vi "Main2.vi"() -> ()   [LabVIEW 2013]
uses:
  controls/Microprobe Vars.ctl
  <userlib>/SweepParameters.ctl
  controls/State.ctl
  controls/ProgramState.ctl
  <instrlib>/Watlow EZ-ZONE/Public/Watlow_Set_Parameter.ctl
  <instrlib>/IMS stepper motors/Address.ctl
  <instrlib>/IMS stepper motors/Set Parameter.ctl
  controls/ProgramColumn.ctl
panel:
  in  "Probe Target State":T1 {"Tset" format="%.1f"; "Telem" format="%.1f"; "GasC" format="%.1f"; "GasB" format="%.1f"; "GasA" format="%.1f"; "Z" format="%.3g"; "Y" format="%.3g"; "X" format="%.3g"; "RampRate" format="%.1f"}
  out "Probe Current State":T1 {"Tset" format="%.1f"; "Telem" format="%.1f"; "GasC" format="%.1f"; "GasB" format="%.1f"; "GasA" format="%.1f"; "Z" format="%.3g"; "Y" format="%.3g"; "X" format="%.3g"; "RampRate" format="%.1f"}
  in  "Exit":bool
  in  "Tab Control":T2(tab)
  in  "Gas B pO2":dbl=0.001
  in  "Gas A pO2":dbl=0.2
  in  "Sample name":string="ZDC30TG3"
  in  "Impedance analyzer":refnum<visa-resource-name>="GPIB0::17::INSTR"
  out "Test sequence path":path
  out "Log file path":path
  out "Sample directory":path
  in  "Motor":refnum<visa-resource-name>="COM9"
  in  "Temp controller":refnum<visa-resource-name>="COM3"
  in  "MFCs":refnum<visa-resource-name>="COM5"
  in  "Inert MFC address":i32=8
  in  "Active MFC address":i32=7
  in  "Instrument type":T3(ring)=enum."BioLogic SP-300"
  out "Estimated pO2":dbl
  in  "Set current as origin":bool
  out "Temperature vs time":dbl(graph)
  in  "Jog to Y":dbl format="%.3g"
  in  "Jog to X":dbl format="%.3g"
  in  "Jog":bool
  out "Chiller flow?":bool
  out "Gases vs time":cluster{"GasA":dbl, "GasB":dbl, "GasC":dbl}(graph)
  out "State":T4
  in  "Run program":bool
  in  "Program":string[][](table)
  in  "Read program":bool
  out "Program data":dbl[][](array[numeric])
  out "Cur step":i32
  in  "Start step":i32=1
  out "Number of steps":i32
  out "Est. time":dbl
  out "Program state":T5
  out "Waiting":dbl
  in  "Take single AC Scan":bool
  in  "Sweep Parameters":T6={"Frequency steps"=41, "Sweep Direction"=enum."Down", "Max frequency (Hz)"=1000000.0, "Min frequency (Hz)"=100.0, "Voltage Level (V)"=0.03, "bias(V)"=0.0} {"Voltage Level (V)" min=0.005 max=20.0 step=0.001 format="%.4f"; "Min frequency (Hz)" format="%#_6e"; "Max frequency (Hz)" format="%#_6e"}
  out "Impedance plot":cluster{dbl[], dbl[]}(graph)
  in  "check if\ntouching\nparams":T6={"Frequency steps"=6, "Sweep Direction"=enum."Down", "Max frequency (Hz)"=1000.0, "Min frequency (Hz)"=100.0, "Voltage Level (V)"=0.03, "bias(V)"=0.0} {"Voltage Level (V)" min=0.005 max=20.0 step=0.001 format="%.4f"; "Min frequency (Hz)" format="%#_6e"; "Max frequency (Hz)" format="%#_6e"}
  out "error out":errorcluster
  out "Monitoring error":errorcluster
  out "State machine error":errorcluster
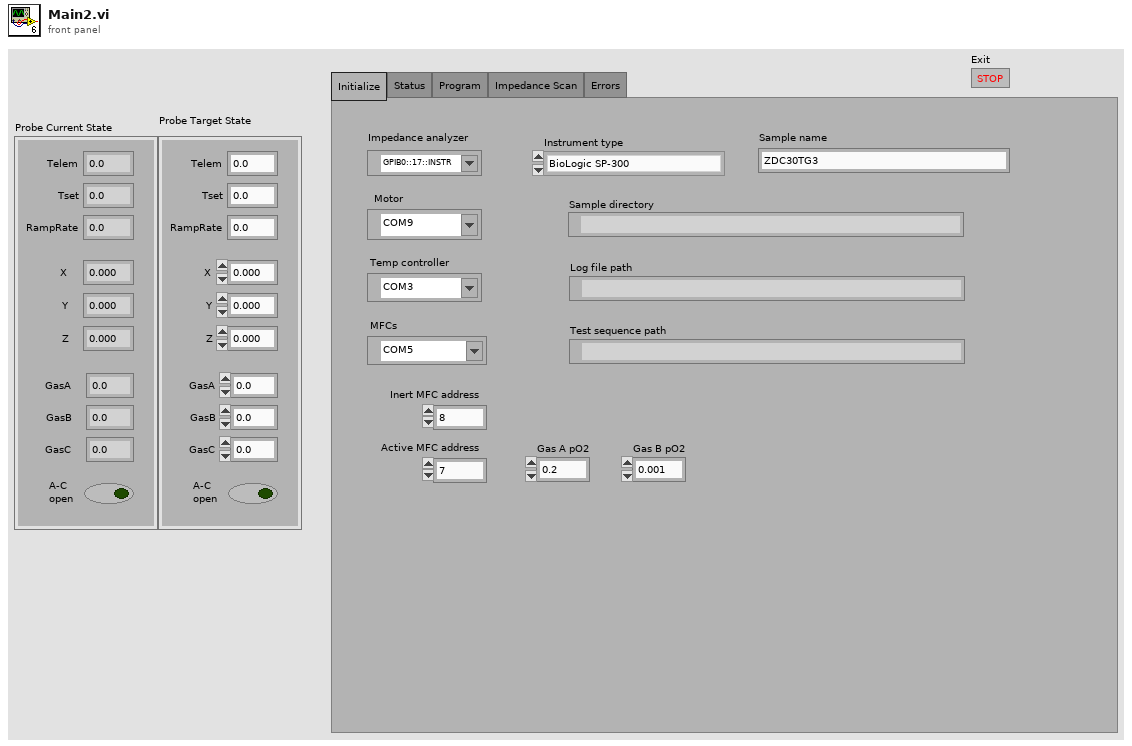
[diagram p1: front panel]
types:
  T1 = typedef "Microprobe Vars.ctl" = cluster{"Telem":dbl, "Tset":dbl, "RampRate":dbl, "X":dbl, "Y":dbl, "Z":dbl, "GasA":dbl, "GasB":dbl, "GasC":dbl, "A-C\nopen":bool}
  T2 = enum32{"Initialize", "Status", "Program", "Impedance Scan", "Errors"}
  T3 = enum16{"Agilent 4285A", "Solartron 1260", "BioLogic SP-300"}
  T4 = typedef "State.ctl" = enum16{"Idle", "Jog", "Run AC Scan", "Run Program", "Exit"}
  T5 = typedef "ProgramState.ctl" = enum16{"Lift Z", "Read program", "Set gas", "Set temperature", "Wait for temperature", "Delay", "Check if running", "Move to position", "Check if touching", "Wait for measurement", "Take measurement", "Move away", "Move to next step?"}
  T6 = typedef "SweepParameters.ctl" = cluster{"Frequency steps":i32, "Sweep Direction":enum16{"Down", "Up"}, "Max frequency (Hz)":dbl, "Min frequency (Hz)":dbl, "Voltage Level (V)":dbl, "bias(V)":dbl}
  T7 = typedef "Watlow_Set_Parameter.ctl" = enum16{"Setpoint", "Ramp Rate", "Setpoint Min", "Setpoint Max"}
  T8 = typedef "Address.ctl" = enum16{"X", "Y", "Z"}
  T9 = typedef "Set Parameter.ctl" = enum16{"Acceleration (A)", "Baud Rate (BD)", "Counter 1 (C1)", "Counter 2 (C2)", "Control C Software Reset (CE)", "Check Sum Enable (CK)", "Clock Mode (CM)", "Clock Mode Ratio (CR)", "Clock Mode Out Step Width (CW)", "Deceleration (D)", "Digital Filtering, Input 1 (D1)", "Digital Filtering, Input 2 (D2)", "Digital Filtering, Input 3 (D3)", "Digital Filtering, Input 4 (D4)", "Digital Filtering, Input 5 (D5)", "Digital Filtering, Input 9 (D9)", "Digital Filtering, Input 10 (D10)", "Digital Filtering, Input 11 (D11)", "Digital Filtering, Input 12 (D12)", "Deadband (DB)", "Decrement Variable (DC)", "Enable/Disable Drive (DE)", "Device Name (DN)", "End Program Execution (E)", "Encoder Function Enable (EE)", "Encoder Lines (EL)", "Echo Mode (EM)", "Escape (ES)", "Execute Program at Address (EX)", "Hold (H)", "Hold Current (HC)", "Hold Current Delay Time (HI)", "Home to Encoder Index (HM)", "Home to Home Switch (HT)", "Increment Variable (IC)", "Initialize Parameters to NVM (IP)", "Input into Variable (IV)", "Jog Enable (JE)", "Limit Stop Mode (LM)", "Move Absolute (MA)", "Move Relative (MR)", "MicroStepping Select (MS)", "Motor Settling Delay Time (MT)", "Output 1 (O1)", "Output 2 (O2)", "Output 3 (O3)", "Output 4 (O4)", "Output 9 (O9)", "Output 10 (O10)", "Output 11 (O11)", "Output 12 (O12)", "Output High Byte (9-12) (OH)", "Output Low Byte (1-4) (OL)", "Output Total (1-4 and 9-12) (OT)", "Position Maintenance (PM)", "Party Mode (PY)", "Register 1 (R1)", "Register 2 (R2)", "Register 3 (R3)", "Register 4 (R4)", "Run Current (RC)", "SetupLimits (S1,S2)", "Stall Factor (SF)", "Slew (SL)", "Stall Mode Set (SM)", "Upgrade Firmware (UG)", "Velocity Initial (VI)", "Velocity Maximum (VM)"}
  T10 = typedef "ProgramColumn.ctl" = enum16{"Run Number", "Stage Temperature", "Ramp Rate", "Wait", "Gas A", "Gas B", "Gas C", "Row index I", "Column index J", "X position", "Y position", "Z position", "Voltage", "Highest frequency", "Lowest frequency", "Number of freq pts", "Delay", "Move this step?", "bias(V)"}
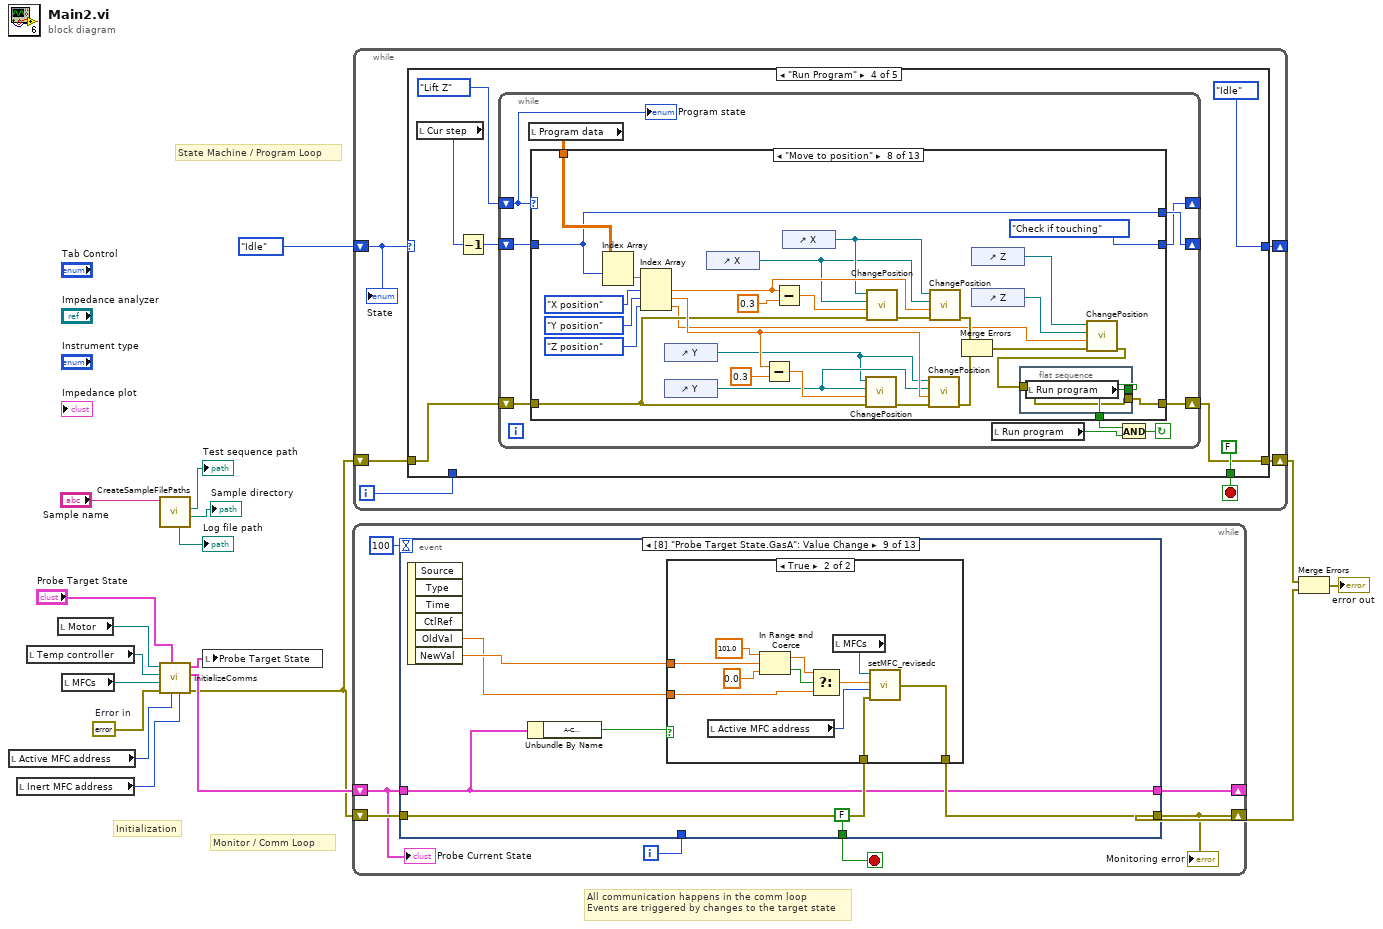
[diagram p0: block diagram]
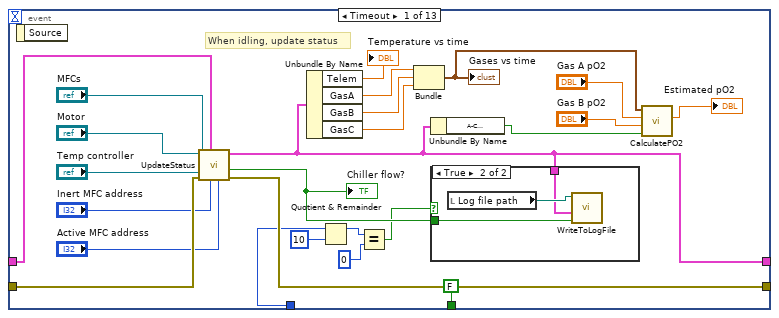
[diagram p2: hidden frame]
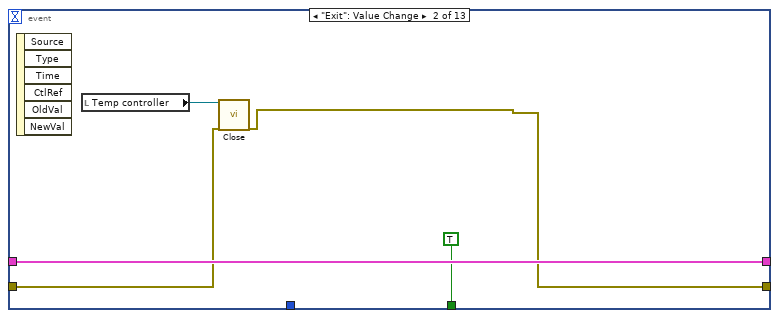
[diagram p4: hidden frame]
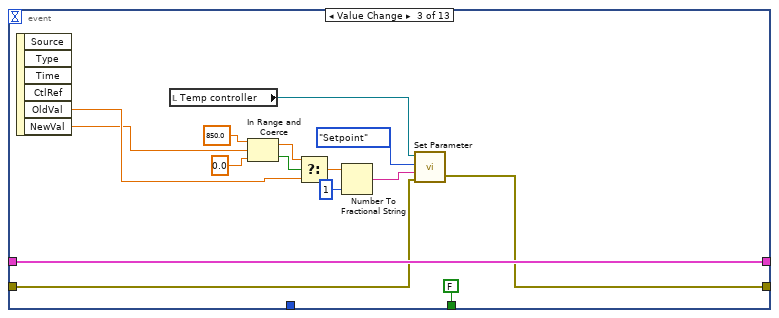
[diagram p5: hidden frame]
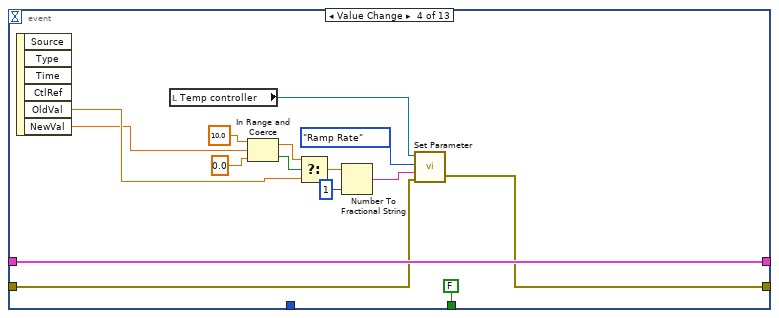
[diagram p6: hidden frame]
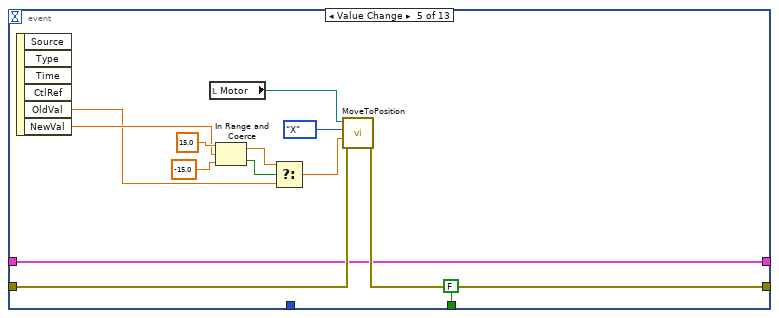
[diagram p7: hidden frame]
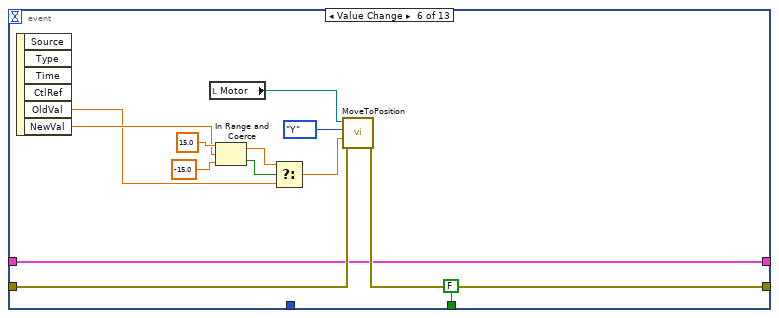
[diagram p8: hidden frame]
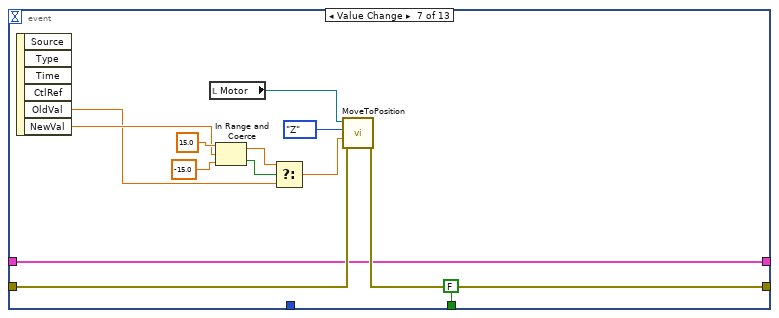
[diagram p9: hidden frame]
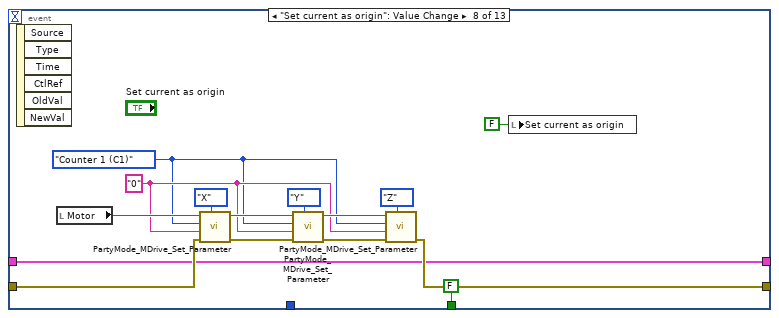
[diagram p10: hidden frame]
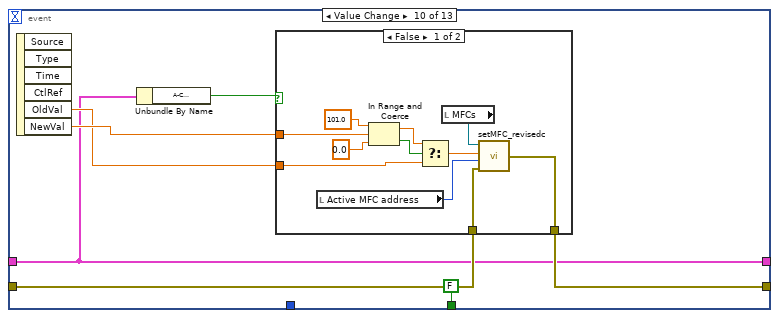
[diagram p12: hidden frame]
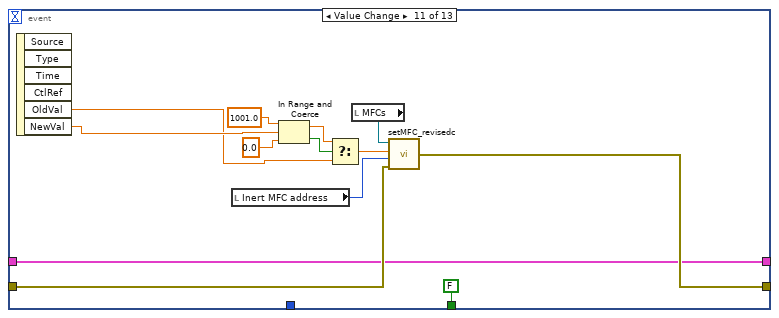
[diagram p14: hidden frame]
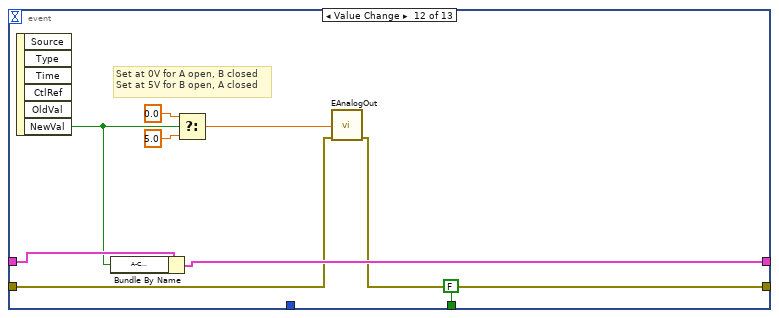
[diagram p15: hidden frame]
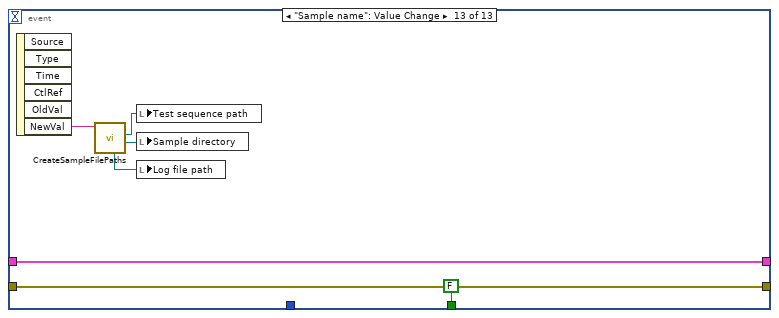
[diagram p16: hidden frame]
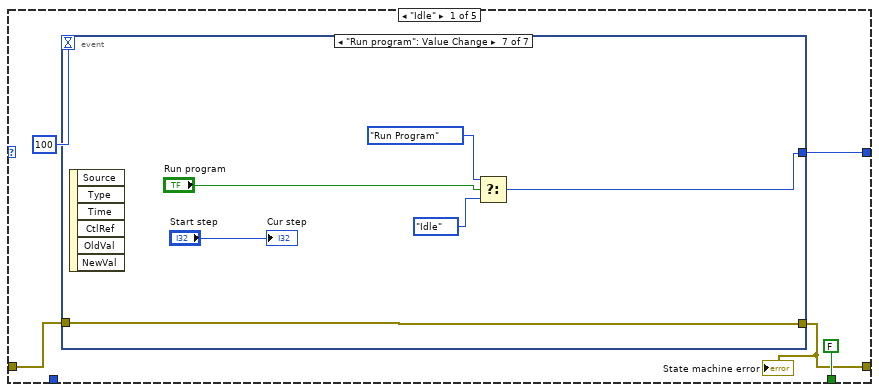
[diagram p17: hidden frame]
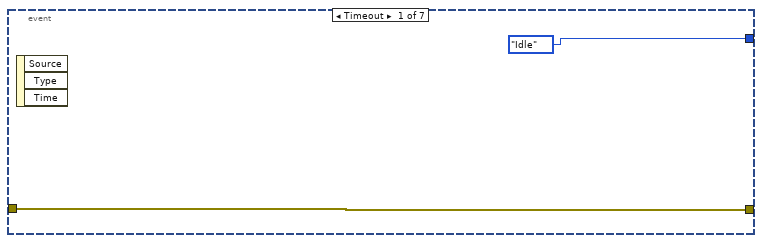
[diagram p18: hidden frame]
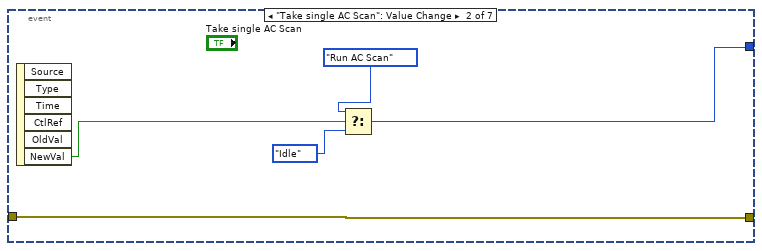
[diagram p19: hidden frame]
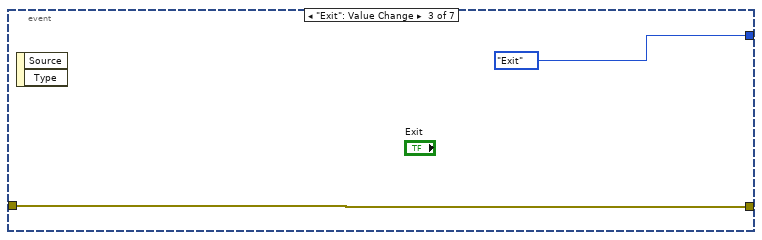
[diagram p20: hidden frame]
diagram:
  w3 = errorcluster {"status"=FALSE, "code"=0, "source"=""}  # Error in
  # "All communication happens in the comm loop\nEvents are triggered by changes to the target state"
  # "Initialization"
  # "State Machine / Program Loop"
  # "Monitor / Comm Loop"
  n1 = local read "Active MFC address"() -> (w8:i32)
  n2 = local read "Inert MFC address"() -> (w7:i32)
  n3 = local read "Temp controller"() -> (w10:refnum<visa-resource-name>)
  n4 = local read "Motor"() -> (w11:refnum<visa-resource-name>)
  n5 = local read "MFCs"() -> (w9:refnum<visa-resource-name>)
  n6 = call "CreateSampleFilePaths.vi"("Sample name"="Sample name") -> ("Sample directory path"=→"Sample directory":path, "Test sequence path"=→"Test sequence path":path, "Log file path"=→"Log file path":path)  [unwired: 8 in]
  n7 = call "InitializeComms.vi"("Inert MFC Channel"=w7, "Active MFC Channel"=w8, "Probe Target State"="Probe Target State", "error in"=w3, "MFC channel"=w9, "Watlow channel"=w10, "Motor channel"=w11) -> ("error out"=w1:errorcluster, "Current probe state"=w6:T1, "Probe Target State out"=w4:T1)  [unwired: 2 in]
  n8 = local write "Probe Target State"(w4) -> ()
  n9 = while {
    shift-right: [w22] -> _
    shift-left: w6 -> [w23]
    shift-right: [w24] -> w16
    shift-left: w1 -> [w25]
    i -> [w19]
    stop <- w20 stop-if-true
    n10 = event shown="[8] \"Probe Target State.GasA\": Value Change" {
      selector: _ -> [_ _ _ _ _ _ _ _ _ _ _ _ _]
      dyn-events: _ -> [_ _ _ _ _ _ _ _ _ _ _ _ _]
      timeout: 100 -> [_ _ _ _ _ _ _ _ _ _ _ _ _]
      tunnel: w25 -> [w46 w56 w61 w76 w100 w113 w126 w141 w147 w166 w185 w195 w205]
      tunnel: [w43 w54 w60 w75 w99 w112 w125 w135 w146 w165 w184 w194 w205] -> w24
      tunnel: w23 -> [w45 w58 w72 w87 w98 w111 w124 w134 w145 w164 w183 w200 w209]
      tunnel: [w32 w58 w72 w87 w98 w111 w124 w134 w145 w164 w183 w199 w209] -> w22
      tunnel: [FALSE TRUE FALSE FALSE FALSE FALSE FALSE FALSE FALSE FALSE FALSE FALSE FALSE] -> w20
      tunnel: w19 -> [w36 _ _ _ _ _ _ _ _ _ _ _ _]
      event Timeout {
        # "When idling, update status"
        n11 = event-data() -> ()  [unwired: 1 in, 1 out]
        n12 = call "UpdateStatus.vi"("Active MFC address"="Active MFC address", "Inert MFC address"="Inert MFC address", "Probe Current State"=w45, "error in"=w46, "MFC Channel"="MFCs", "Watlow channel"="Temp controller", "Motor channel"="Motor") -> ("error out"=w43:errorcluster, "Chiller flow?"=w38:bool, "Updated probe state"=w32:T1)  [unwired: 2 in]
        "Chiller flow?" <- w38
        n13 = Unbundle By Name(w32) -> ("Telem"=→"Temperature vs time":dbl, "GasA"=w40:dbl, "GasB"=w31:dbl, "GasC"=w39:dbl)
        n14 = Quotient & Remainder(x=w36, y=10) -> (x-y*floor(x/y)=w33:i32)  [unwired: 1 out]
        n15 = Equal?(x=w33, y=0) -> (x = y?=w37:bool)
        n16 = Bundle("GasA"=w40, "GasB"=w31, "GasC"=w39) -> (w26:cluster{"GasA":dbl, "GasB":dbl, "GasC":dbl})  [unwired: 1 in]
        "Gases vs time" <- w26
        n17 = Unbundle By Name(w32) -> ("A-C\nopen"=w30:bool)
        n18 = case shown="True" w37 {
          tunnel: w32 -> [_ w52]
          tunnel: w38 -> [_ w51]
          frame False {
          }
          frame True {
            n19 = local read "Log file path"() -> (w53:path)
            n20 = call <instrlib>:"WriteToLogFile.vi"("Chiller flow?"=w51, "Probe Current State"=w52, "file path (dialog if empty)"=w53) -> ()  [unwired: 9 in]
          }
        }
        n21 = call "CalculatePO2.vi"("A-C open"=w30, "Gas B pO2"="Gas B pO2", "Gas A pO2"="Gas A pO2", "Gases vs time"=w26) -> ("Estimated pO2"=→"Estimated pO2":dbl)  [unwired: 7 in]
      }
      event "Exit": Value Change {
        n22 = event-data() -> ()  [unwired: 1 in, 6 out]
        n23 = local read "Temp controller"() -> (w55:refnum<visa-resource-name>)
        n24 = call <instrlib>:"Close.vi"("PC Comms Port"=w55, "Error In"=w56) -> ("Error Out"=w54:errorcluster)  [unwired: 16 in, 1 out]
      }
      event Value Change {
        n25 = event-data() -> ("OldVal"=w63:dbl, "NewVal"=w62:dbl)  [unwired: 1 in, 4 out]
        n26 = local read "Temp controller"() -> (w59:refnum<visa-resource-name>)
        n27 = In Range and Coerce(upper limit=850.0, x=w62, lower limit=0.0) -> (coerced(x)=w71:dbl, In Range?=w66:bool)
        n28 = Select(t=w71, s=w66, f=w63) -> (s? t:f=w70:dbl)
        n29 = Number To Fractional String(number=w70, precision (6)=i16 1) -> (F-format string=w69:string)  [unwired: 2 in]
        n30 = call <instrlib>:"Set Parameter.vi"("Error In"=w61, "Set Parameter"=Watlow_Set_Parameter."Setpoint", "Write Value"=w69, "PC Comms Port"=w59) -> ("Error Out"=w60:errorcluster)  [unwired: 1 out]
      }
      event Value Change {
        n31 = event-data() -> ("OldVal"=w78:dbl, "NewVal"=w77:dbl)  [unwired: 1 in, 4 out]
        n32 = local read "Temp controller"() -> (w74:refnum<visa-resource-name>)
        n33 = In Range and Coerce(upper limit=10.0, x=w77, lower limit=0.0) -> (coerced(x)=w86:dbl, In Range?=w81:bool)
        n34 = Select(t=w86, s=w81, f=w78) -> (s? t:f=w85:dbl)
        n35 = Number To Fractional String(number=w85, precision (6)=i16 1) -> (F-format string=w84:string)  [unwired: 2 in]
        n36 = call <instrlib>:"Set Parameter.vi"("Error In"=w76, "Set Parameter"=Watlow_Set_Parameter."Ramp Rate", "Write Value"=w84, "PC Comms Port"=w74) -> ("Error Out"=w75:errorcluster)  [unwired: 1 out]
      }
      event Value Change {
        n37 = event-data() -> ("OldVal"=w91:dbl, "NewVal"=w94:dbl)  [unwired: 1 in, 4 out]
        n38 = local read "Motor"() -> (w89:refnum<visa-resource-name>)
        n39 = In Range and Coerce(upper limit=15.0, x=w94, lower limit=-15.0) -> (coerced(x)=w92:dbl, In Range?=w93:bool)
        n40 = Select(t=w92, s=w93, f=w91) -> (s? t:f=w90:dbl)
        n41 = call <instrlib>:"MoveToPosition.vi"("error out 2"=w100, "Position"=w90, "Address"=Address."X", "Motor channel"=w89) -> ("error out"=w99:errorcluster)  [unwired: 5 in, 2 out]
      }
      event Value Change {
        n42 = event-data() -> ("OldVal"=w104:dbl, "NewVal"=w107:dbl)  [unwired: 1 in, 4 out]
        n43 = local read "Motor"() -> (w102:refnum<visa-resource-name>)
        n44 = In Range and Coerce(upper limit=15.0, x=w107, lower limit=-15.0) -> (coerced(x)=w105:dbl, In Range?=w106:bool)
        n45 = Select(t=w105, s=w106, f=w104) -> (s? t:f=w103:dbl)
        n46 = call <instrlib>:"MoveToPosition.vi"("error out 2"=w113, "Position"=w103, "Address"=Address."Y", "Motor channel"=w102) -> ("error out"=w112:errorcluster)  [unwired: 5 in, 2 out]
      }
      event Value Change {
        n47 = event-data() -> ("OldVal"=w117:dbl, "NewVal"=w120:dbl)  [unwired: 1 in, 4 out]
        n48 = local read "Motor"() -> (w115:refnum<visa-resource-name>)
        n49 = In Range and Coerce(upper limit=15.0, x=w120, lower limit=-15.0) -> (coerced(x)=w118:dbl, In Range?=w119:bool)
        n50 = Select(t=w118, s=w119, f=w117) -> (s? t:f=w116:dbl)
        n51 = call <instrlib>:"MoveToPosition.vi"("error out 2"=w126, "Position"=w116, "Address"=Address."Z", "Motor channel"=w115) -> ("error out"=w125:errorcluster)  [unwired: 5 in, 2 out]
      }
      event "Set current as origin": Value Change {
        w132 = Set_Parameter."Counter 1 (C1)" ("Set Parameter")
        w133 = "0" ("Parameter Setpoint")
        n52 = event-data() -> ()  [unwired: 1 in, 6 out]
        n53 = local read "Motor"() -> (w138:refnum<visa-resource-name>)
        n54 = call <instrlib>:"PartyMode_MDrive_Set_Parameter.vi"("Address"=Address."X", "error out 2"=w141, "Parameter Setpoint"=w133, "Set Parameter"=w132, "VISA resource name out 2"=w138) -> ("error out"=w140:errorcluster, "VISA resource name out"=w137:refnum<visa-resource-name>)  [unwired: 1 in, 1 out]
        n55 = call <instrlib>:"PartyMode_MDrive_Set_Parameter.vi"("Address"=Address."Y", "error out 2"=w140, "Parameter Setpoint"=w133, "Set Parameter"=w132, "VISA resource name out 2"=w137) -> ("error out"=w136:errorcluster, "VISA resource name out"=w139:refnum<visa-resource-name>)  [unwired: 1 in, 1 out]
        n56 = call <instrlib>:"PartyMode_MDrive_Set_Parameter.vi"("Address"=Address."Z", "error out 2"=w136, "Parameter Setpoint"=w133, "Set Parameter"=w132, "VISA resource name out 2"=w139) -> ("error out"=w135:errorcluster)  [unwired: 1 in, 2 out]
        n57 = local write "Set current as origin"(FALSE ("Set current as origin")) -> ()
      }
      event Value Change {
        n58 = event-data() -> ("OldVal"=w148:dbl, "NewVal"=w149:dbl)  [unwired: 1 in, 4 out]
        n59 = Unbundle By Name(w145) -> ("A-C\nopen"=w144:bool)
        n60 = case shown="True" w144 {
          tunnel: w149 -> [_ w152]
          tunnel: w148 -> [_ w157]
          tunnel: w147 -> [w150 w155]
          tunnel: [w150 w154] -> w146
          frame False {
          }
          frame True {
            n61 = local read "Active MFC address"() -> (w153:i32)
            n62 = In Range and Coerce(upper limit=101.0, x=w152, lower limit=0.0) -> (coerced(x)=w161:dbl, In Range?=w160:bool)
            n63 = Select(t=w161, s=w160, f=w157) -> (s? t:f=w156:dbl)
            n64 = local read "MFCs"() -> (w151:refnum<visa-resource-name>)
            n65 = call <instrlib>:"setMFC_revisedc.vi"("error in (no error)"=w155, "channel"=w153, "Set Flow Rate sccm"=w156, "VISA resource name"=w151) -> ("error out"=w154:errorcluster)
          }
        }
      }
      event Value Change {
        n66 = event-data() -> ("OldVal"=w167:dbl, "NewVal"=w168:dbl)  [unwired: 1 in, 4 out]
        n67 = Unbundle By Name(w164) -> ("A-C\nopen"=w163:bool)
        n68 = case shown="False" w163 {
          tunnel: w168 -> [w170 _]
          tunnel: w167 -> [w175 _]
          tunnel: w166 -> [w173 w180]
          tunnel: [w172 w180] -> w165
          frame False {
            n69 = local read "Active MFC address"() -> (w171:i32)
            n70 = In Range and Coerce(upper limit=101.0, x=w170, lower limit=0.0) -> (coerced(x)=w179:dbl, In Range?=w178:bool)
            n71 = Select(t=w179, s=w178, f=w175) -> (s? t:f=w174:dbl)
            n72 = local read "MFCs"() -> (w169:refnum<visa-resource-name>)
            n73 = call <instrlib>:"setMFC_revisedc.vi"("error in (no error)"=w173, "channel"=w171, "Set Flow Rate sccm"=w174, "VISA resource name"=w169) -> ("error out"=w172:errorcluster)
          }
          frame True {
          }
        }
      }
      event Value Change {
        n74 = event-data() -> ("OldVal"=w186:dbl, "NewVal"=w187:dbl)  [unwired: 1 in, 4 out]
        n75 = local read "Inert MFC address"() -> (w193:i32)
        n76 = In Range and Coerce(upper limit=1001.0, x=w187, lower limit=0.0) -> (coerced(x)=w188:dbl, In Range?=w189:bool)
        n77 = Select(t=w188, s=w189, f=w186) -> (s? t:f=w192:dbl)
        n78 = local read "MFCs"() -> (w181:refnum<visa-resource-name>)
        n79 = call <instrlib>:"setMFC_revisedc.vi"("error in (no error)"=w185, "channel"=w193, "Set Flow Rate sccm"=w192, "VISA resource name"=w181) -> ("error out"=w184:errorcluster)
      }
      event Value Change {
        # "Set at 0V for A open, B closed\nSet at 5V for B open, A closed"
        n80 = event-data() -> ("NewVal"=w198:bool)  [unwired: 1 in, 5 out]
        n81 = Bundle By Name(cluster=w200, "A-C\nopen"=w198) -> (w199:T1)
        n82 = Select(t=0.0, s=w198, f=5.0) -> (s? t:f=w196:dbl)
        n83 = call <vilib>:"EAnalogOut.vi"("Analog Output 0 [volts]"=w196, "error in"=w195) -> ("error out"=w194:errorcluster)  [unwired: 12 in, 1 out]
      }
      event "Sample name": Value Change {
        n84 = event-data() -> ("NewVal"=w204:string)  [unwired: 1 in, 5 out]
        n85 = call "CreateSampleFilePaths.vi"("Sample name"=w204) -> ("Sample directory path"=w207:path, "Test sequence path"=w208:path, "Log file path"=w206:path)  [unwired: 8 in]
        n86 = local write "Test sequence path"(w208) -> ()
        n87 = local write "Sample directory"(w207) -> ()
        n88 = local write "Log file path"(w206) -> ()
      }
    }
    "Monitoring error" <- w24
    "Probe Current State" <- w23
  }
  n89 = while {
    shift-right: [w211] -> w17
    shift-left: w1 -> [w214]
    shift-right: [w213] -> _
    shift-left: State."Idle" ("States") -> [w215]
    i -> [w210]
    stop <- w212 stop-if-true
    n90 = case shown="\"Run Program\"" w215 {
      tunnel: w214 -> [w219 w267 w287 w315 w623]
      tunnel: [w216 w254 w276 w314 w623] -> w211
      tunnel: [w220 State."Idle" ("States") State."Idle" ("States") State."Idle" ("States") State."Exit" ("States")] -> w213
      tunnel: [FALSE FALSE FALSE FALSE TRUE] -> w212
      tunnel: w210 -> [_ _ w286 _ _]
      frame "Idle" {
        n91 = event shown="[6] \"Run program\": Value Change" {
          selector: _ -> [_ _ _ _ _ _ _]
          dyn-events: _ -> [_ _ _ _ _ _ _]
          timeout: 100 -> [_ _ _ _ _ _ _]
          tunnel: [State."Idle" ("States") w223 State."Exit" ("States") w231 State."Idle" ("States") State."Idle" ("States") w248] -> w220
          tunnel: w219 -> [w221 w227 w228 w232 w237 w244 w253]
          tunnel: [w221 w227 w228 w232 w236 w244 w253] -> w216
          event Timeout {
            n92 = event-data() -> ()  [unwired: 1 in, 3 out]
          }
          event "Take single AC Scan": Value Change {
            n93 = event-data() -> ("NewVal"=w226:bool)  [unwired: 1 in, 5 out]
            n94 = Select(t=State."Run AC Scan" ("States"), s=w226, f=State."Idle" ("States")) -> (s? t:f=w223:T4)
          }
          event "Exit": Value Change {
            n95 = event-data() -> ()  [unwired: 1 in, 2 out]
          }
          event "Jog": Value Change {
            n96 = event-data() -> ()  [unwired: 1 in, 6 out]
            n97 = case shown="True" "Jog" {
              tunnel: [State."Idle" ("States") State."Jog" ("States")] -> w231
              frame False {
              }
              frame True {
              }
            }
          }
          event "Read program": Value Change {
            n98 = event-data() -> ()  [unwired: 1 in, 6 out]
            n99 = local read "Test sequence path"() -> (w241:path)
            n100 = call "ReadProgramData.vi"("error in (no error)"=w237, "file path (dialog if empty)"=w241) -> ("error out"=w236:errorcluster, "Number of steps"=→"Number of steps":i32, "Program data"=→"Program data":dbl[][], "Program"=w235:string[][], "Est. time"=→"Est. time":dbl)  [unwired: 5 in]
            n101 = local write "Program"(w235) -> ()
          }
          event "Program": Value Change {
            n102 = event-data() -> ("NewVal"=w245:string[][])  [unwired: 1 in, 5 out]
            n103 = Decimal String To Number(string=w245, default (0L)=0.0) -> (number=w246:dbl[][])  [unwired: 1 in, 1 out]
            n104 = local write "Program data"(w246) -> ()
          }
          event "Run program": Value Change {
            n105 = event-data() -> ()  [unwired: 1 in, 6 out]
            n106 = Select(t=State."Run Program" ("States"), s="Run program", f=State."Idle" ("States")) -> (s? t:f=w248:T4)
            "Cur step" <- "Start step"
          }
        }
        "State machine error" <- w216
      }
      frame "Jog" {
        # "To register a \"Value Change\" event to move motors\nuse references. Also use references to retrieve current values"
        # "Current"
        # "Targets"
        n107 = control-ref of="X"() -> (w264:refnum<vi>)
        n108 = control-ref of="Z"() -> (w262:refnum<vi>)
        n109 = control-ref of="Y"() -> (w263:refnum<vi>)
        n110 = Build Array(w264, w263, w262) -> (w261:refnum<vi>[])
        n111 = control-ref of="Z"() -> (w258:refnum<vi>)
        n112 = control-ref of="X"() -> (w260:refnum<vi>)
        n113 = control-ref of="Y"() -> (w259:refnum<vi>)
        n114 = Build Array(w260, w259, w258) -> (w257:refnum<vi>[])
        n115 = call <instrlib>:"JogToPosition.vi"("Target position refs"=w261, "Current position refs"=w257, "Jog to X"="Jog to X", "Jog to Y"="Jog to Y", "error out 2"=w267) -> ("error in 2"=w255:errorcluster)  [unwired: 10 in]
        n116 = case shown="No Error" w255 {
          selector: w255 -> [w269 w271]
          tunnel: [w269 w271] -> w254
          frame No Error {
            n117 = local write "Jog"(FALSE ("Jog")) -> ()
          }
          frame Error {
          }
        }
      }
      frame "Run AC Scan" {
        n118 = local read "Sample directory"() -> (w285:path)
        n119 = local read "Impedance analyzer"() -> (w272:refnum<visa-resource-name>)
        n120 = local read "Instrument type"() -> (w275:T3)
        n121 = Number To Decimal String(number=w286) -> (decimal integer string=w280:string)  [unwired: 1 in]
        n122 = Path to Array of Strings(0:w285) -> (2:w284:string[])  [unwired: 1 out]
        n123 = Concatenate Strings("SCAN", w280, ".txt" ("string")) -> (w278:string)
        n124 = Build Array (concatenate)(w284, w278) -> (w283:string[])
        n125 = Array of Strings to Path(0:w283) -> (2:w282:path)  [unwired: 1 in]
        n126 = control-ref of="Impedance plot"() -> (w273:refnum<vi>)
        n127 = case shown="\"BioLogic SP-300\"" w275 {
          tunnel: w287 -> [w295 w297 w307]
          tunnel: w282 -> [w294 w299 w304]
          tunnel: [w293 w296 w306] -> w277
          tunnel: "Sweep Parameters" -> [w292 w300 w305]
          tunnel: w273 -> [w291 w298 w302]
          tunnel: w272 -> [w290 w301 _]
          frame "Agilent 4285A", Default {
            n128 = call <instrlib>:"Agilent 4285A Series Frequency Sweep.vi"("Impedance plot reference"=w291, "file path (dialog if empty)"=w294, "Sweep parameters"=w292, "Agilent 4285A Channel"=w290, "error in (no error)"=w295) -> ("error out"=w293:errorcluster)  [unwired: 8 in, 2 out]
          }
          frame "Solartron 1260" {
            n129 = call <instrlib>:"S1260RecycleSweep.vi"("VISA resource name"=w301, "Impedance plot reference"=w298, "file path (dialog if empty)"=w299, "Sweep Parameters"=w300, "error in (no error)"=w297) -> ("error out"=w296:errorcluster)  [unwired: 8 in, 2 out]
          }
          frame "BioLogic SP-300" {
            n130 = call "peis_CK.vi"("Nyquist plot reference"=w302, "error in (no error)"=w307, "Sweep Parameters"=w305, "file path (dialog if empty)"=w304, "IP adress"="192.109.209.128") -> ("error out"=w306:errorcluster)  [unwired: 5 in, 1 out]
          }
        }
        n131 = case shown="No Error" w277 {
          selector: w277 -> [w308 w310]
          tunnel: [w308 w310] -> w276
          frame No Error {
            n132 = local write "Take single AC Scan"(FALSE ("Take single AC Scan")) -> ()
          }
          frame Error {
            n133 = local write "Take single AC Scan"(FALSE ("Take single AC Scan")) -> ()
          }
        }
      }
      frame "Run Program" {
        n134 = local read "Cur step"() -> (w313:i32)
        n135 = Decrement(x=w313) -> (x-1=w312:i32)
        n136 = while {
          shift-right: [w321] -> _
          shift-left: w312 -> [w326]
          shift-right: [w325] -> w314
          shift-left: w315 -> [w327]
          shift-right: [w320] -> _
          shift-left: ProgramState."Lift Z" ("Program state") -> [w328]
          stop <- w324 continue-if-true
          n137 = local read "Program data"() -> (w319:dbl[][])
          n138 = case shown="\"Move to position\"" w328 {
            tunnel: w319 -> [w339 _ w378 w392 w402 w423 w439 w470 _ w533 w570 w602 w615]
            tunnel: w327 -> [w336 w354 w371 w381 w400 w421 w441 w456 w474 w531 w559 w594 w607]
            tunnel: w326 -> [w331 w356 w370 w388 w398 w418 w438 w469 w475 w528 w552 w598 w605]
            tunnel: [w335 w353 w359 w382 w397 w420 w441 w443 w476 w530 w558 w593 w607] -> w325
            tunnel: [w331 w356 w370 w388 w398 w418 w438 w469 w475 w528 w552 w598 w608] -> w321
            tunnel: [ProgramState."Read program" ("Program state") ProgramState."Set gas" ("Program state") ProgramState."Set temperature" ("Program state") ProgramState."Wait for temperature" ("Program state") ProgramState."Delay" ("Program state") ProgramState."Check if running" ("Program state") w433 ProgramState."Check if touching" ("Program state") ProgramState."Wait for measurement" ("Program state") ProgramState."Take measurement" ("Program state") w545 ProgramState."Move to next step?" ("Program state") ProgramState."Read program" ("Program state")] -> w320
            tunnel: [TRUE ("Run program") TRUE ("Run program") TRUE ("Run program") TRUE ("Run program") TRUE ("Run program") TRUE ("Run program") w440 w442 w473 w526 TRUE ("Run program") TRUE ("Run program") w606] -> w322
            frame "Lift Z", Default {
              n139 = Index Array(array=w339, index (row) #1=w331, index (col) #1=ProgramColumn."Z position" ("Enum"), index (row) #2=w331, index (col) #2=ProgramColumn."Move this step?" ("Enum")) -> (element #1=w337:dbl, element #2=w330:dbl)
              n140 = Not Equal To 0?(x=w330) -> (x != 0?=w329:bool)
              n141 = case shown="True" w329 {
                tunnel: w337 -> [_ w347]
                tunnel: w336 -> [w340 w342]
                tunnel: [w340 w341] -> w335
                frame False {
                }
                frame True {
                  n142 = control-ref of="Z"() -> (w345:refnum<vi>)
                  n143 = control-ref of="Z"() -> (w344:refnum<vi>)
                  n144 = Subtract(x=w347, y=0.3) -> (x-y=w343:dbl)
                  n145 = call "ChangePosition.vi"("error in (no error)"=w342, "Target value"=w343, "Actual ref"=w344, "Target ref"=w345) -> ("error out"=w341:errorcluster)  [unwired: 7 in]
                }
              }
            }
            frame "Read program" {
              n146 = local read "Test sequence path"() -> (w355:path)
              n147 = call "ReadProgramData.vi"("error in (no error)"=w354, "file path (dialog if empty)"=w355) -> ("error out"=w353:errorcluster, "Number of steps"=w348:i32, "Program data"=w349:dbl[][], "Program"=w350:string[][], "Est. time"=w351:dbl)  [unwired: 5 in]
              n148 = local write "Number of steps"(w348) -> ()
              n149 = local write "Est. time"(w351) -> ()
              n150 = local write "Program data"(w349) -> ()
              n151 = local write "Program"(w350) -> ()
            }
            frame "Set gas" {
              n152 = Index Array(array=w378, index (row)=w370) -> (element=w377:dbl[])  [unwired: 1 in]
              n153 = Index Array(array=w377, index #1=ProgramColumn."Gas A" ("Enum"), index #2=ProgramColumn."Gas B" ("Enum"), index #3=ProgramColumn."Gas C" ("Enum")) -> (element #1=w367:dbl, element #2=w366:dbl, element #3=w365:dbl)
              n154 = control-ref of="A-C\nopen"() -> (w373:refnum<vi>)
              n155 = Greater?(x=w367, y=w366) -> (0:w372:bool)
              n156 = property class="Bool (strict)"(reference=w373, error in=w371, "Val(Sgnl)"=w372) -> (error out=w362:errorcluster)  [unwired: 1 out]
              n157 = control-ref of="GasA"() -> (w368:refnum<vi>)
              n158 = property class="DigNum (strict)"(reference=w368, error in=w362, "Val(Sgnl)"=w367) -> (error out=w361:errorcluster)  [unwired: 1 out]
              n159 = control-ref of="GasB"() -> (w364:refnum<vi>)
              n160 = property class="DigNum (strict)"(reference=w364, error in=w361, "Val(Sgnl)"=w366) -> (error out=w360:errorcluster)  [unwired: 1 out]
              n161 = control-ref of="GasC"() -> (w363:refnum<vi>)
              n162 = property class="DigNum (strict)"(reference=w363, error in=w360, "Val(Sgnl)"=w365) -> (error out=w359:errorcluster)  [unwired: 1 out]
            }
            frame "Set temperature" {
              n163 = Index Array(array=w392, index (row)=w388) -> (element=w391:dbl[])  [unwired: 1 in]
              n164 = Index Array(array=w391, index #1=ProgramColumn."Ramp Rate" ("Enum"), index #2=ProgramColumn."Stage Temperature" ("Enum")) -> (element #1=w386:dbl, element #2=w385:dbl)
              n165 = Greater?(x=w386, y=w385) -> ()  [unwired: 1 out]
              n166 = control-ref of="RampRate"() -> (w380:refnum<vi>)
              n167 = property class="DigNum (strict)"(reference=w380, error in=w381, "Val(Sgnl)"=w386) -> (error out=w384:errorcluster)  [unwired: 1 out]
              n168 = control-ref of="Tset"() -> (w379:refnum<vi>)
              n169 = property class="DigNum (strict)"(reference=w379, error in=w384, "Val(Sgnl)"=w385) -> (error out=w382:errorcluster)  [unwired: 1 out]
            }
            frame "Wait for temperature" {
              n170 = Index Array(array=w402, index (row)=w398) -> (element=w401:dbl[])  [unwired: 1 in]
              n171 = control-ref of="Telem"() -> (w394:refnum<vi>)
              n172 = Index Array(array=w401, index=ProgramColumn."Stage Temperature" ("Enum")) -> (element=w395:dbl)
              n173 = while {
                tunnel: w394 -> [w413]
                shift-right: [w412] -> w397
                shift-left: w400 -> [w407]
                tunnel: w395 -> [w406]
                stop <- w403 continue-if-true
                n174 = property class="DigNum (strict)"(reference=w413, error in=w407) -> (error out=w412:errorcluster, "Value"=w411:dbl)  [unwired: 1 out]
                n175 = local read "Run program"() -> (w405:bool)
                n176 = Subtract(x=w406, y=w411) -> (x-y=w410:dbl)
                n177 = Absolute Value(x=w410) -> (abs(x)=w409:dbl)
                n178 = Greater?(x=w409, y=5.0) -> (0:w404:bool)
                n179 = And(x=w404, y=w405) -> (x .and. y?=w403:bool)
              }
            }
            frame "Delay" {
              n180 = Index Array(array=w423, index (row)=w418, index (col)=ProgramColumn."Wait" ("Enum")) -> (element=w417:dbl)
              n181 = Multiply(x=w417, y=60.0) -> (x*y=w415:dbl)
              n182 = while {
                shift-right: [w427] -> _
                shift-left: w415 -> [w430]
                shift-right: [w426] -> w420
                shift-left: w421 -> [w426]
                stop <- w428 continue-if-true
                n183 = local read "Run program"() -> (w425:bool)
                n184 = Subtract(x=w430, y=1.0) -> (x-y=w427:dbl)
                n185 = Wait (ms)(milliseconds to wait=u32 1000) -> ()  [unwired: 1 out]
                n186 = Greater Than 0?(x=w427) -> (x > 0?=w424:bool)
                n187 = And(x=w425, y=w424) -> (x .and. y?=w428:bool)
                "Waiting" <- w430
              }
            }
            frame "Check if running" {
              n188 = Index Array(array=w439, index (row)=w438, index (col)=ProgramColumn."Move this step?" ("Enum")) -> (element=w432:dbl)
              n189 = local read "Run program"() -> (w440:bool)
              n190 = Not Equal To 0?(x=w432) -> (x != 0?=w435:bool)
              n191 = Select(t=ProgramState."Move to position" ("Program state"), s=w435, f=ProgramState."Wait for measurement" ("Program state")) -> (s? t:f=w433:T5)
            }
            frame "Move to position" {
              n192 = Index Array(array=w470, index (row)=w469) -> (element=w467:dbl[])  [unwired: 1 in]
              n193 = Index Array(array=w467, index #1=ProgramColumn."X position" ("Enum"), index #2=ProgramColumn."Y position" ("Enum"), index #3=ProgramColumn."Z position" ("Enum")) -> (element #1=w455:dbl, element #2=w458:dbl, element #3=w445:dbl)
              n194 = control-ref of="Y"() -> (w450:refnum<vi>)
              n195 = control-ref of="Y"() -> (w451:refnum<vi>)
              n196 = control-ref of="X"() -> (w452:refnum<vi>)
              n197 = Subtract(x=w458, y=0.3) -> (x-y=w457:dbl)
              n198 = Subtract(x=w455, y=0.3) -> (x-y=w454:dbl)
              n199 = control-ref of="X"() -> (w453:refnum<vi>)
              n200 = call "ChangePosition.vi"("error in (no error)"=w456, "Target value"=w457, "Actual ref"=w451, "Target ref"=w450) -> ("error out"=w462:errorcluster)  [unwired: 7 in]
              n201 = call "ChangePosition.vi"("error in (no error)"=w456, "Target value"=w454, "Actual ref"=w452, "Target ref"=w453) -> ("error out"=w461:errorcluster)  [unwired: 7 in]
              n202 = call "ChangePosition.vi"("error in (no error)"=w462, "Target value"=w458, "Actual ref"=w451, "Target ref"=w450) -> ("error out"=w463:errorcluster)  [unwired: 7 in]
              n203 = call "ChangePosition.vi"("error in (no error)"=w461, "Target value"=w455, "Actual ref"=w452, "Target ref"=w453) -> ("error out"=w464:errorcluster)  [unwired: 7 in]
              n204 = Merge Errors(w464, w463) -> (w449:errorcluster)
              n205 = control-ref of="Z"() -> (w448:refnum<vi>)
              n206 = control-ref of="Z"() -> (w447:refnum<vi>)
              n207 = flat-sequence {
                tunnel: [w472] -> w442
                tunnel: w444 -> [w471]
                tunnel: [w471] -> w443
                frame #0 {
                  n208 = local read "Run program"() -> (w472:bool)
                }
              }
              n209 = call "ChangePosition.vi"("error in (no error)"=w449, "Target value"=w445, "Actual ref"=w447, "Target ref"=w448) -> ("error out"=w444:errorcluster)  [unwired: 7 in]
            }
            frame "Check if touching" {
              n210 = while {
                tunnel: w474 -> [w492]
                tunnel: [w485] -> w476
                tunnel: [w478] -> w473
                i -> [w491]
                stop <- w478 stop-if-true
                n211 = local read "Impedance analyzer"() -> (w482:refnum<visa-resource-name>)
                n212 = local read "Instrument type"() -> (w493:T3)
                n213 = control-ref of="Impedance plot"() -> (w484:refnum<vi>)
                n214 = case shown="\"BioLogic SP-300\"" w493 {
                  tunnel: w492 -> [w507 w515 w521]
                  tunnel: [w511 w514 w523] -> w486
                  tunnel: [w508 w513 w522] -> w489
                  tunnel: w484 -> [w506 w512 w524]
                  tunnel: "check if\ntouching\nparams" -> [w505 w516 w520]
                  tunnel: w482 -> [w504 w517 _]
                  frame "Agilent 4285A", Default {
                    n215 = String To Path(string="") -> (path=w509:path)
                    n216 = call <instrlib>:"Agilent 4285A Series Frequency Sweep.vi"("Impedance plot reference"=w506, "file path (dialog if empty)"=w509, "Sweep parameters"=w505, "Agilent 4285A Channel"=w504, "error in (no error)"=w507) -> ("Impedance data"=w508:dbl[][], "error out"=w511:errorcluster)  [unwired: 8 in, 1 out]
                  }
                  frame "Solartron 1260" {
                    n217 = String To Path(string="") -> (path=w518:path)
                    n218 = call <instrlib>:"S1260RecycleSweep.vi"("VISA resource name"=w517, "Impedance plot reference"=w512, "file path (dialog if empty)"=w518, "Sweep Parameters"=w516, "error in (no error)"=w515) -> ("Impedance data"=w513:dbl[][], "error out"=w514:errorcluster)  [unwired: 8 in, 1 out]
                  }
                  frame "BioLogic SP-300" {
                    n219 = call "peis_CK.vi"("Nyquist plot reference"=w524, "error in (no error)"=w521, "Sweep Parameters"=w520, "IP adress"="192.109.209.128") -> ("error out"=w523:errorcluster, "impedance data"=w522:dbl[][])  [unwired: 6 in]
                  }
                }
                n220 = call "IsProbeTouchingDot"("array"=w489) -> ("Within range"=w487:bool)  [unwired: 10 in]
                n221 = Greater Or Equal?(x=w491, y=5) -> (x >= y?=w488:bool)
                n222 = Or(x=w488, y=w487) -> (x .or. y?=w479:bool)
                n223 = case shown="False" w487 {
                  tunnel: w486 -> [w502 w503]
                  tunnel: [w498 w503] -> w485
                  frame False {
                    n224 = control-ref of="Z"() -> (w494:refnum<vi>)
                    n225 = property class="DigNum (strict)"(reference=w494, error in=w502) -> (reference out=w499:refnum<vi>, error out=w497:errorcluster, "Value"=w501:dbl)
                    n226 = control-ref of="Z"() -> (w495:refnum<vi>)
                    n227 = Add(x=w501, y=0.005) -> (x+y=w496:dbl)
                    n228 = call "ChangePosition.vi"("error in (no error)"=w497, "Target value"=w496, "Actual ref"=w495, "Target ref"=w499) -> ("error out"=w498:errorcluster)  [unwired: 7 in]
                  }
                  frame True {
                  }
                }
                n229 = local read "Run program"() -> (w481:bool)
                n230 = Not(x=w481) -> (.not. x?=w480:bool)
                n231 = Or(x=w479, y=w480) -> (x .or. y?=w478:bool)
              }
            }
            frame "Wait for measurement" {
              n232 = Index Array(array=w533, index (row)=w528, index (col)=ProgramColumn."Delay" ("Enum")) -> (element=w527:dbl)
              n233 = while {
                shift-right: [w537] -> _
                shift-left: w527 -> [w540]
                shift-right: [w536] -> w530
                shift-left: w531 -> [w536]
                tunnel: [w534] -> w526
                stop <- w538 continue-if-true
                n234 = local read "Run program"() -> (w534:bool)
                n235 = Subtract(x=w540, y=1.0) -> (x-y=w537:dbl)
                n236 = Wait (ms)(milliseconds to wait=u32 1000) -> ()  [unwired: 1 out]
                n237 = Greater Than 0?(x=w537) -> (x > 0?=w535:bool)
                n238 = And(x=w534, y=w535) -> (x .and. y?=w538:bool)
              }
            }
            frame "Take measurement" {
              n239 = Index Array(array=w570, index (row)=w552) -> (element=w550:dbl[])  [unwired: 1 in]
              n240 = Index Array(array=w550, index #1=ProgramColumn."Number of freq pts" ("Enum"), index #2=ProgramColumn."Highest frequency" ("Enum"), index #3=ProgramColumn."Lowest frequency" ("Enum"), index #4=ProgramColumn."Voltage" ("Enum"), index #5=ProgramColumn."Move this step?" ("Enum"), index #6=ProgramColumn."bias(V)" ("Enum")) -> (element #1=w569:dbl, element #2=w568:dbl, element #3=w567:dbl, element #4=w566:dbl, element #5=w547:dbl, element #6=w543:dbl)
              n241 = Bundle By Name(cluster=T6 {"Frequency steps"=11, "Sweep Direction"=enum."Down", "Max frequency (Hz)"=100000.0, "Min frequency (Hz)"=100.0, "Voltage Level (V)"=0.03, "bias(V)"=0.0} ("Sweep Parameters 2"), "Frequency steps"=w569, "Sweep Direction"=enum16{"Down", "Up"}."Down", "Max frequency (Hz)"=w568, "Min frequency (Hz)"=w567, "Voltage Level (V)"=w566, "bias(V)"=w543) -> (w560:T6)
              n242 = local read "Sample directory"() -> (w554:path)
              n243 = local read "Program"() -> (w553:string[][])
              n244 = local read "Instrument type"() -> (w571:T3)
              n245 = local read "Impedance analyzer"() -> (w556:refnum<visa-resource-name>)
              n246 = control-ref of="Impedance plot"() -> (w555:refnum<vi>)
              n247 = call "MakeScanFilename.vi"("Program"=w553, "index (row)"=w552, "Sample directory"=w554) -> ("path"=w551:path)  [unwired: 8 in]
              n248 = case shown="\"BioLogic SP-300\"" w571 {
                tunnel: w560 -> [w578 w580 w590]
                tunnel: w559 -> [w577 w581 w587]
                tunnel: [w576 w582 w586] -> w558
                tunnel: w556 -> [w575 w584 _]
                tunnel: w555 -> [w574 w579 w588]
                tunnel: w551 -> [w573 w583 w589]
                frame "Agilent 4285A", Default {
                  n249 = call <instrlib>:"Agilent 4285A Series Frequency Sweep.vi"("Impedance plot reference"=w574, "file path (dialog if empty)"=w573, "Sweep parameters"=w578, "Agilent 4285A Channel"=w575, "error in (no error)"=w577) -> ("error out"=w576:errorcluster)  [unwired: 8 in, 2 out]
                }
                frame "Solartron 1260" {
                  n250 = call <instrlib>:"S1260RecycleSweep.vi"("VISA resource name"=w584, "Impedance plot reference"=w579, "file path (dialog if empty)"=w583, "Sweep Parameters"=w580, "error in (no error)"=w581) -> ("error out"=w582:errorcluster)  [unwired: 8 in, 2 out]
                }
                frame "BioLogic SP-300" {
                  n251 = call "peis_CK.vi"("Nyquist plot reference"=w588, "error in (no error)"=w587, "Sweep Parameters"=w590, "file path (dialog if empty)"=w589, "IP adress"="192.109.209.128") -> ("error out"=w586:errorcluster)  [unwired: 5 in, 1 out]
                }
              }
              n252 = Not Equal To 0?(x=w547) -> (x != 0?=w546:bool)
              n253 = Select(t=ProgramState."Move away" ("Program state"), s=w546, f=ProgramState."Move to next step?" ("Program state")) -> (s? t:f=w545:T5)
            }
            frame "Move away" {
              n254 = Index Array(array=w602, index (row)=w598, index (col)=ProgramColumn."Z position" ("Enum")) -> (element=w600:dbl)
              n255 = control-ref of="Z"() -> (w597:refnum<vi>)
              n256 = control-ref of="Z"() -> (w596:refnum<vi>)
              n257 = Subtract(x=w600, y=0.3) -> (x-y=w595:dbl)
              n258 = call "ChangePosition.vi"("error in (no error)"=w594, "Target value"=w595, "Actual ref"=w596, "Target ref"=w597) -> ("error out"=w593:errorcluster)  [unwired: 7 in]
            }
            frame "Move to next step?" {
              n259 = Increment(x=w605) -> (x+1=w609:i32)
              n260 = local read "Number of steps"() -> (w604:i32)
              n261 = Index Array(array=w615, index (row)=w609) -> (element=w614:dbl[])  [unwired: 1 in]
              n262 = Array Max & Min(array=w614) -> (max value=w613:dbl, min value=w612:dbl)  [unwired: 2 out]
              n263 = Equal?(x=w613, y=w612) -> (x = y?=w611:bool)
              n264 = Greater?(x=w605, y=w604) -> (0:w603:bool)
              n265 = Or(x=w603, y=w611) -> (x .or. y?=w610:bool)
              n266 = case shown="False" w610 {
                tunnel: w609 -> [w617 _]
                tunnel: [w617 w620] -> w608
                tunnel: [TRUE ("Run program") w621] -> w606
                frame False {
                  n267 = Increment(x=w617) -> (x+1=w618:i32)
                  n268 = local write "Cur step"(w618) -> ()
                }
                frame True {
                  w620 = 0
                  w621 = FALSE ("Run program")
                  n269 = local write "Run program"(w621) -> ()
                  n270 = local write "Cur step"(w620) -> ()
                }
              }
            }
          }
          n271 = local read "Run program"() -> (w323:bool)
          n272 = And(x=w322, y=w323) -> (x .and. y?=w324:bool)
          "Program state" <- w328
        }
      }
      frame "Exit" {
      }
    }
    "State" <- w215
  }
  n273 = Merge Errors(w17, w16) -> (→"error out":errorcluster)
